vi "convert to pumps.vi"(11 "control values":dbl[](array[numeric])) -> (0 "minimum pulse time (ms) 2":u32, 3 "Control out":T1 {"Pumps"."0 to 1" format="%.2f"; "Pumps"."flow rate" format="%.2f"})   [LabVIEW 2015]
uses:
  Stamp 2 control.ctl
  Peristaltic/Pump w direction.ctl
  mini peristaltic pump.ctl
  Pump Direction.ctl
  3-stop colors and numbers.ctl
panel:
  out "subarray":dbl[](array[numeric])
  in  "Control":T1={"Switches"=[FALSE, FALSE, FALSE, FALSE, FALSE, FALSE, FALSE, FALSE, FALSE, FALSE, FALSE, FALSE, FALSE], "Pumps"=[{"on/off"=FALSE, "Direction"=FALSE, "flow rate"=0.0, "Tubing"=enum."orange-black", "tubing or 0 to 1"=FALSE, "0 to 1"=0.0}, {"on/off"=FALSE, "Direction"=FALSE, "flow rate"=0.0, "Tubing"=enum."orange-black", "tubing or 0 to 1"=FALSE, "0 to 1"=0.0}, {"on/off"=FALSE, "Direction"=FALSE, "flow rate"=0.0, "Tubing"=enum."orange-black", "tubing or 0 to 1"=FALSE, "0 to 1"=0.0}, {"on/off"=FALSE, "Direction"=FALSE, "flow rate"=0.0, "Tubing"=enum."orange-black", "tubing or 0 to 1"=FALSE, "0 to 1"=0.0}, {"on/off"=FALSE, "Direction"=FALSE, "flow rate"=0.0, "Tubing"=enum."orange-black", "tubing or 0 to 1"=FALSE, "0 to 1"=0.0}, {"on/off"=FALSE, "Direction"=FALSE, "flow rate"=0.0, "Tubing"=enum."orange-black", "tubing or 0 to 1"=FALSE, "0 to 1"=0.0}]} {"Pumps"."0 to 1" format="%.2f"; "Pumps"."flow rate" format="%.2f"}
  # "0-12"
  # "0-12"
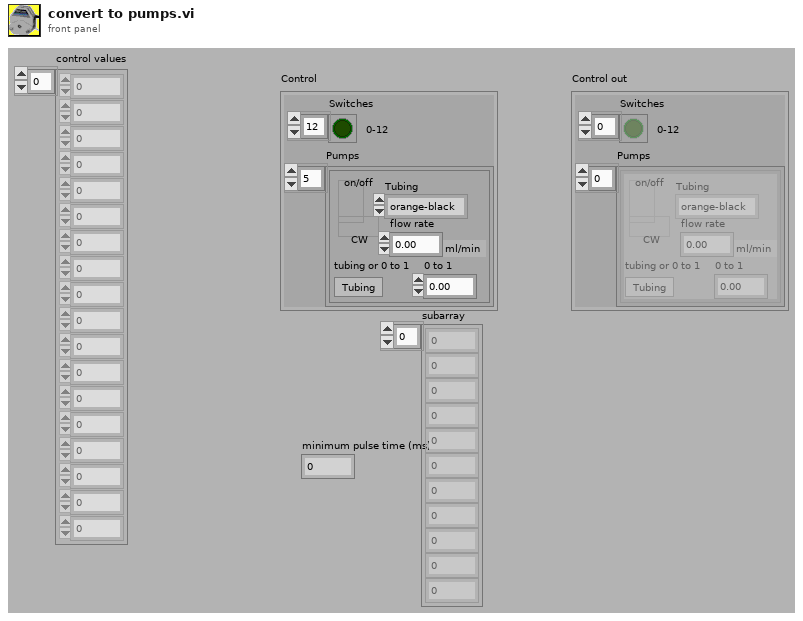
[diagram p1: front panel]
types:
  T1 = typedef "Stamp 2 control.ctl" = cluster{"Switches":bool[], "Pumps":T2[]}
  T2 = typedef "Pump w direction.ctl" = cluster{"on/off":T3, "Direction":T4, "flow rate":dbl[unit], "Tubing":T5, "tubing or 0 to 1":bool, "0 to 1":dbl}
  T3 = typedef "mini peristaltic pump.ctl" = bool
  T4 = typedef "Pump Direction.ctl" = bool
  T5 = typedef "3-stop colors and numbers.ctl" = enum16{"orange-black", "orange-red", "orange-blue", "orange-green", "green-yellow", "orange-yellow", "white-yellow", "orange-white", "black-black", "orange-orange", "white-black", "white-white", "white-red", "red-red", "red-grey", "grey-grey", "yellow-yellow", "yellow-blue", "blue-blue", "blue-green", "green-green", "purple-purple", "purple-black", "purple-orange", "purple-white", "black-white", "13", "14", "15", "16", "17", "18"}
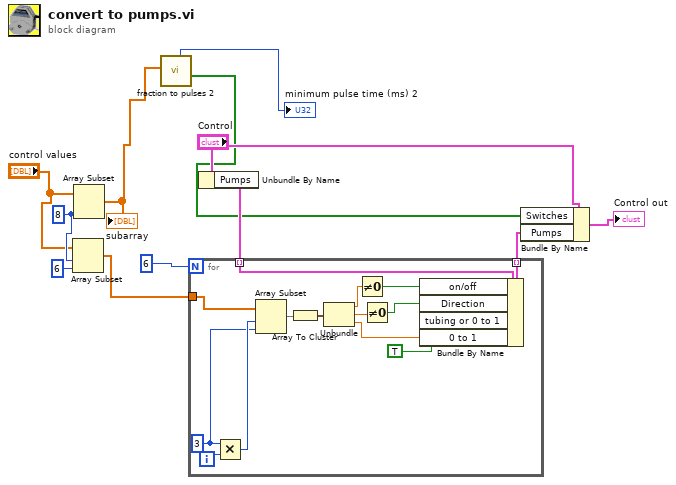
[diagram p0: block diagram]
diagram:
  w10 = 8 ("length")
  n1 = Array Subset(array="control values", index=w10, length=6) -> (w5:dbl[])
  n2 = Array Subset(array="control values", length=w10) -> (w3:dbl[])  [unwired: 1 in]
  "subarray" <- w3
  n3 = call "fraction to pulses 2.vi"("fractions"=w3) -> ("switch state"=w2:bool[], "minimum pulse time (ms) 2"=→"minimum pulse time (ms) 2":u32)  [unwired: 5 in, 4 out]
  n4 = Unbundle By Name("Control") -> ("Pumps"=w7:T2[])
  n5 = for {
    N: 6 -> [_]
    tunnel: w7 -> [w26] mode=indexing
    tunnel: [w25] -> w6 mode=indexing
    tunnel: w5 -> [w22]
    i -> [w23]
    w20 = 3 ("x")
    n6 = Multiply(x=w20, y=w23) -> (x*y=w21:i32)
    n7 = Array Subset(array=w22, index=w21, length=w20) -> (w19:dbl[])
    n8 = Array To Cluster(array=w19) -> (cluster=w18:cluster{"[0]":dbl, "[1]":dbl, "[2]":dbl})
    n9 = Unbundle(w18) -> ("[0]"=w17:dbl, "[1]"=w15:dbl, "[2]"=w13:dbl)
    n10 = Not Equal To 0?(x=w17) -> (x != 0?=w16:bool)
    n11 = Not Equal To 0?(x=w15) -> (x != 0?=w14:bool)
    n12 = Bundle By Name(cluster=w26, "on/off"=w16, "Direction"=w14, "tubing or 0 to 1"=TRUE, "0 to 1"=w13) -> (w25:T2)
  }
  n13 = Bundle By Name(cluster="Control", "Switches"=w2, "Pumps"=w6) -> (→"Control out":T1)
